vi "Interrupts.vi"(2 "AnalogTriggers":T3[](array[typedef])=[{"InHysteresis"=FALSE, "OverLimit"=FALSE, "Rising"=FALSE, "Falling"=FALSE}, {"InHysteresis"=FALSE, "OverLimit"=FALSE, "Rising"=FALSE, "Falling"=FALSE}, {"InHysteresis"=FALSE, "OverLimit"=FALSE, "Rising"=FALSE, "Falling"=FALSE}, {"InHysteresis"=FALSE, "OverLimit"=FALSE, "Rising"=FALSE, "Falling"=FALSE}, {"InHysteresis"=FALSE, "OverLimit"=FALSE, "Rising"=FALSE, "Falling"=FALSE}, {"InHysteresis"=FALSE, "OverLimit"=FALSE, "Rising"=FALSE, "Falling"=FALSE}, {"InHysteresis"=FALSE, "OverLimit"=FALSE, "Rising"=FALSE, "Falling"=FALSE}, {"InHysteresis"=FALSE, "OverLimit"=FALSE, "Rising"=FALSE, "Falling"=FALSE}], 3 "SystemTime":u32, 4 "DigitalInputs":bool[](array[boolean])=[FALSE, FALSE, FALSE, FALSE, FALSE, FALSE, FALSE, FALSE, FALSE, FALSE, FALSE, FALSE, FALSE, FALSE, FALSE, FALSE, FALSE, FALSE, FALSE, FALSE, FALSE, FALSE, FALSE, FALSE, FALSE, FALSE, FALSE, FALSE, FALSE, FALSE, FALSE, FALSE], 5 "FallingOccurance":refnum<k4>, 6 "RisingOccurance":refnum<k4>, 7 "Config":T2) -> (0 "FallingTimestamp":u32, 1 "RisingTimestamp":u32)   [LabVIEW 2019]
uses:
  Helpers/AnalogTriggerOutput.ctl
  Helpers/Source.ctl
  <vilib>/rvi/Emulation/niFpgaProcessEmulError.vi
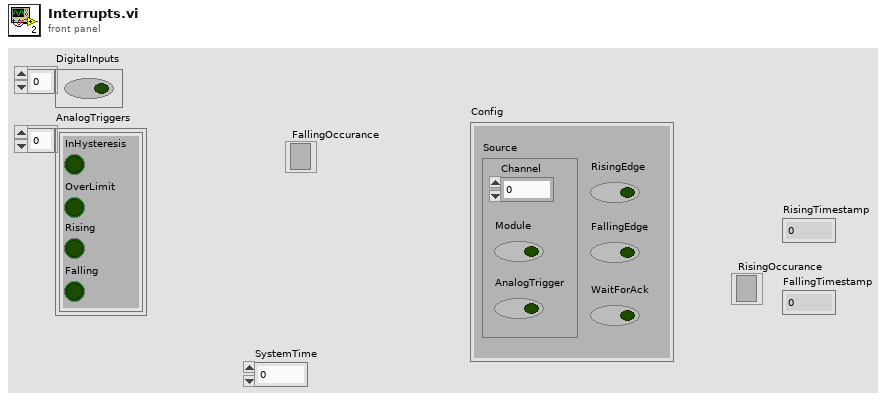
[diagram p1: front panel]
types:
  T1 = typedef "Source.ctl" = cluster{"Channel":fxp<+,4,4>, "Module":bool, "AnalogTrigger":bool}
  T2 = cluster{"Source":T1, "RisingEdge":bool, "FallingEdge":bool, "WaitForAck":bool}
  T3 = typedef "AnalogTriggerOutput.ctl" = cluster{"InHysteresis":bool, "OverLimit":bool, "Rising":bool, "Falling":bool}
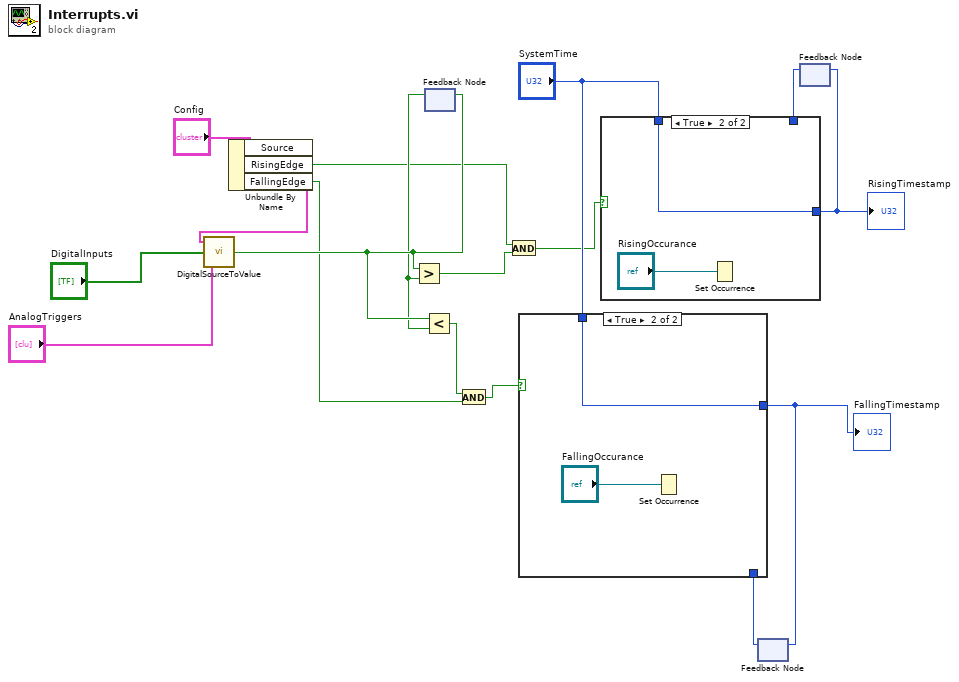
[diagram p0: block diagram]
diagram:
  n1 = Unbundle By Name("Config") -> ("Source"=w7:T1, "RisingEdge"=w5:bool, "FallingEdge"=w2:bool)
  n2 = call "DigitalSourceToValue.vi"("AnalogTriggers"="AnalogTriggers", "DigitalInputs"="DigitalInputs", "Source"=w7) -> ("Value"=w15:bool)
  n3 = feedback-in #1(w15) -> ()
  n4 = feedback #1() -> (w14:bool)  [unwired: 1 in]
  n5 = Greater?(x=w15, y=w14) -> (0:w6:bool)
  n6 = Less?(x=w15, y=w14) -> (x < y?=w3:bool)
  n7 = And(x=w3, y=w2) -> (x .and. y?=w1:bool)
  n8 = And(x=w5, y=w6) -> (x .and. y?=w4:bool)
  n9 = feedback #2() -> (w11:u32)  [unwired: 1 in]
  n10 = case shown="True" w1 {
    tunnel: [w18 w19] -> w12
    tunnel: "SystemTime" -> [_ w19]
    tunnel: w11 -> [w18 _]
    frame False {
    }
    frame True {
      n11 = Set Occurrence("FallingOccurance") -> ()
    }
  }
  "FallingTimestamp" <- w12
  n12 = feedback-in #2(w12) -> ()
  n13 = feedback #3() -> (w9:u32)  [unwired: 1 in]
  n14 = case shown="True" w4 {
    tunnel: "SystemTime" -> [_ w22]
    tunnel: [w21 w22] -> w10
    tunnel: w9 -> [w21 _]
    frame False {
    }
    frame True {
      n15 = Set Occurrence("RisingOccurance") -> ()
    }
  }
  "RisingTimestamp" <- w10
  n16 = feedback-in #3(w10) -> ()
